vi "removeNode.vi"(0 "reference":refnum<class "Graph.lvclass">, 1 "node":refnum<class "AbstractNode.lvclass">, 2 "RemoveChildrenIfAny(False)":bool, 5 "error in (no error)":errorcluster) -> (14 "reference out":refnum<class "Graph.lvclass">, 19 "error out":errorcluster)   [LabVIEW 2016, in "Graph.lvclass"]
doc: "public void removeNode(Node n)"
uses:
  <resource>/Framework/Providers/Open_GDS/UML/Graph_class/Graph.lvclass
  <resource>/Framework/Providers/Open_GDS/UML/AbstractNode_class/AbstractNode.lvclass
  <resource>/Framework/Providers/Open_GDS/UML/PackageNode_class/PackageNode.lvclass
  C:/Program Files (x86)/National Instruments/LabVIEW 2016/resource/Framework/Providers/Open_GDS/UML/AbstractNode_class/AbstractNode.lvclass
  <resource>/Framework/Providers/Open_GDS/UML/AbstractEdge_class/AbstractEdge.lvclass
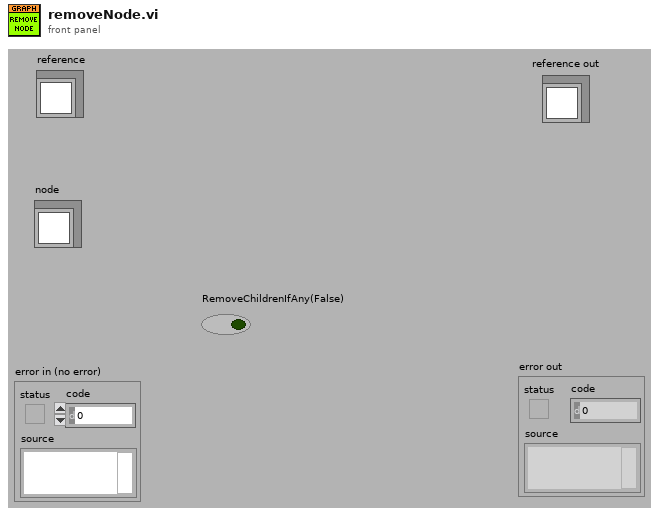
[diagram p1: front panel]
types:
  T1 = typedef "Graph.lvclass/ObjectAttributes.ctl" = cluster{"nodes":refnum<class "AbstractNode.lvclass">[], "edges":refnum<class "AbstractEdge.lvclass">[], "nodesToBeRemoved":refnum<class "AbstractNode.lvclass">[], "edgesToBeRemoved":refnum<class "AbstractEdge.lvclass">[], "needsLayout":bool, "LayoutNodes":refnum<class "AbstractNode.lvclass">[]}
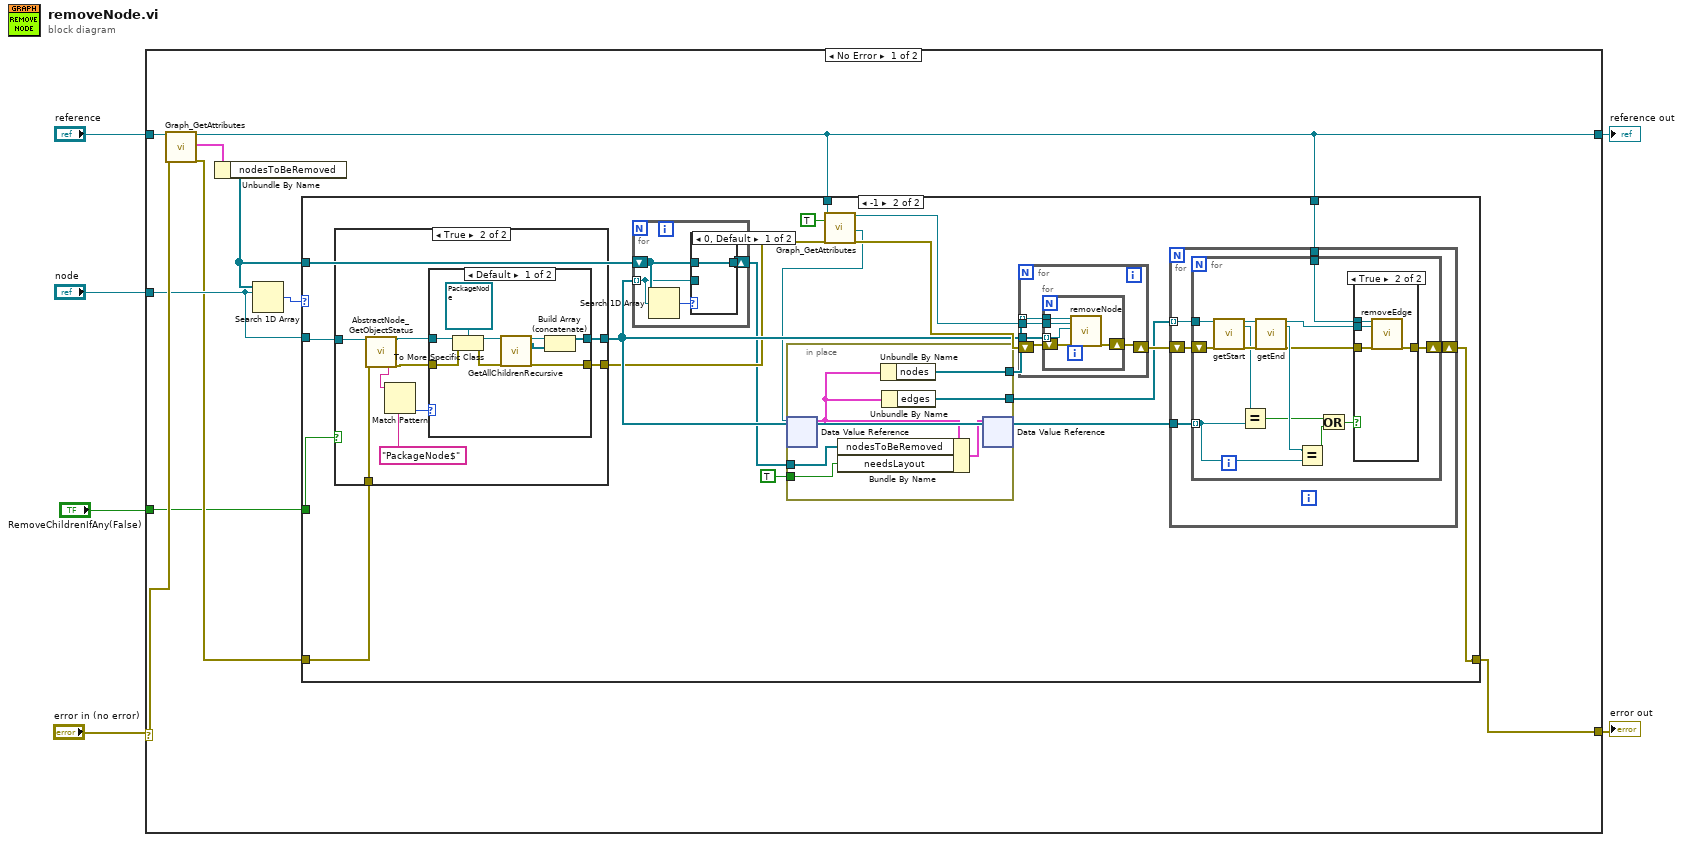
[diagram p0: block diagram]
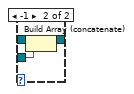
[diagram p3: hidden frame]
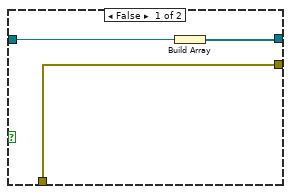
[diagram p4: hidden frame]
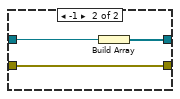
[diagram p5: hidden frame]
diagram:
  n1 = case shown="No Error" "error in (no error)" {
    selector: "error in (no error)" -> [w13 w108]
    tunnel: "reference" -> [w16 w109]
    tunnel: [w15 w108] -> w5
    tunnel: [w14 w109] -> w4
    tunnel: "node" -> [w12 _]
    tunnel: "RemoveChildrenIfAny(False)" -> [w8 _]
    frame No Error {
      n2 = call <resource>:"Graph_GetAttributes.vi"("reference in"=w16, "error in (no error)"=w13) -> ("reference out"=w14:refnum<class "Graph.lvclass">, "Data"=w7:T1, "error out"=w10:errorcluster)  [unwired: 1 in, 14 out]
      n3 = Unbundle By Name(w7) -> ("nodesToBeRemoved"=w9:refnum<class "AbstractNode.lvclass">[])
      n4 = Search 1D Array(1D array=w9, element=w12) -> (index of element=w11:i32)  [unwired: 1 out]
      n5 = case shown="-1" w11 {
        tunnel: w10 -> [w17 w26]
        tunnel: [w17 w30] -> w15
        tunnel: w14 -> [_ w35]
        tunnel: w9 -> [_ w34]
        tunnel: w12 -> [_ w27]
        tunnel: w14 -> [_ w29]
        tunnel: w8 -> [_ w24]
        frame 0, Default {
        }
        frame -1 {
          n6 = case shown="True" w24 {
            tunnel: [w51 w61] -> w28
            tunnel: w27 -> [w52 w60]
            tunnel: w26 -> [w50 w59]
            tunnel: [w50 w54] -> w25
            frame False {
              n7 = Build Array(w52) -> (w51:refnum<class "AbstractNode.lvclass">[])
            }
            frame True {
              n8 = call <resource>:"AbstractNode_GetObjectStatus.vi"("reference in"=w60, "error in (no error)"=w59) -> ("Class name"=w53:string, "reference out"=w56:refnum<class "AbstractNode.lvclass">, "error out"=w55:errorcluster)  [unwired: 15 out]
              n9 = Match Pattern(string=w53, regular expression="PackageNode$" ("y")) -> (offset past match=w57:i32)  [unwired: 4 out]
              n10 = case shown="Default" w57 {
                tunnel: [w62 w72] -> w54
                tunnel: [w63 w71] -> w61
                tunnel: w56 -> [w70 w73]
                tunnel: w55 -> [w68 w72]
                frame Default {
                  n11 = To More Specific Class(target class=refnum<class "PackageNode.lvclass"> refnum ("reference in"), reference=w70, error in=w68) -> (specific class reference=w66:refnum<class "PackageNode.lvclass">, error out=w67:errorcluster)
                  n12 = call <resource>:"GetAllChildrenRecursive.vi"("reference"=w66, "error in (no error)"=w67) -> ("reference out"=w65:refnum<class "PackageNode.lvclass">, "children"=w64:refnum<class "AbstractNode.lvclass">[], "error out"=w62:errorcluster)  [unwired: 15 in]
                  n13 = Build Array (concatenate)(w65, w64) -> (w63:refnum<class "AbstractNode.lvclass">[])
                }
                frame -1 {
                  n14 = Build Array(w73) -> (w71:refnum<class "AbstractNode.lvclass">[])
                }
              }
            }
          }
          n15 = for {
            tunnel: w28 -> [w42] mode=indexing
            shift-right: [w45] -> w19
            shift-left: w34 -> [w44]
            n16 = Search 1D Array(1D array=w44, element=w42) -> (index of element=w43:i32)  [unwired: 1 out]
            n17 = case shown="0, Default" w43 {
              tunnel: [w46 w49] -> w45
              tunnel: w42 -> [_ w48]
              tunnel: w44 -> [w46 w47]
              frame 0, Default {
              }
              frame -1 {
                n18 = Build Array (concatenate)(w47, w48) -> (w49:refnum<class "AbstractNode.lvclass">[])
              }
            }
          }
          n19 = call <resource>:"Graph_GetAttributes.vi"("reference in"=w35, "OnlyGetDvrReference(False)"=TRUE, "error in (no error)"=w25) -> ("reference out"=w33:refnum<class "Graph.lvclass">, "DataRef"=w22:refnum<data-value>, "error out"=w32:errorcluster)  [unwired: 13 in, 1 out]
          n20 = in-place {
            in-place-border: [w40] -> w21
            in-place-border: [w39] -> w20
            in-place-border: w19 -> [w38]
            in-place-border: TRUE ("needsLayout") -> [w37]
            n21 = in-place-dvr #1(w22) -> (w41:T1)  [unwired: 1 out]
            n22 = Bundle By Name(cluster=w41, "nodesToBeRemoved"=w38, "needsLayout"=w37) -> (w36:T1)
            n23 = Unbundle By Name(w41) -> ("nodes"=w40:refnum<class "AbstractNode.lvclass">[])
            n24 = Unbundle By Name(w41) -> ("edges"=w39:refnum<class "AbstractEdge.lvclass">[])
            n25 = in-place-dvr #1(w36) -> ()  [unwired: 2 out]
          }
          n26 = for {
            tunnel: w21 -> [w102] mode=indexing
            tunnel: w33 -> [w101]
            tunnel: w28 -> [w100]
            shift-right: [w98] -> w31
            shift-left: w32 -> [w99]
            n27 = for {
              tunnel: w102 -> [w107]
              tunnel: w101 -> [w106]
              tunnel: w100 -> [w103] mode=indexing
              shift-right: [w104] -> w98
              shift-left: w99 -> [w105]
              n28 = call-dynamic "removeNode.vi"("reference"=w107, "graph"=w106, "node"=w103, "error in (no error)"=w105) -> ("error out"=w104:errorcluster)  [unwired: 14 in, 1 out]
            }
          }
          n29 = for {
            tunnel: w20 -> [w77] mode=indexing
            shift-right: [w75] -> w30
            shift-left: w31 -> [w78]
            tunnel: w28 -> [w76]
            tunnel: w29 -> [w74]
            n30 = for {
              tunnel: w77 -> [w91]
              tunnel: w76 -> [w86] mode=indexing
              tunnel: w74 -> [w80]
              shift-right: [w83] -> w75
              shift-left: w78 -> [w92]
              n31 = call-dynamic "getStart.vi"("reference"=w91, "error in (no error)"=w92) -> ("reference out"=w90:refnum<class "AbstractEdge.lvclass">, "startNode"=w88:refnum<class "AbstractNode.lvclass">, "error out"=w89:errorcluster)  [unwired: 14 in, 1 out]
              n32 = Equal?(x=w88, y=w86) -> (x = y?=w84:bool)
              n33 = call-dynamic "getEnd.vi"("reference"=w90, "error in (no error)"=w89) -> ("reference out"=w79:refnum<class "AbstractEdge.lvclass">, "endNode"=w87:refnum<class "AbstractNode.lvclass">, "error out"=w82:errorcluster)  [unwired: 14 in, 1 out]
              n34 = Equal?(x=w87, y=w86) -> (x = y?=w85:bool)
              n35 = Or(x=w84, y=w85) -> (x .or. y?=w81:bool)
              n36 = case shown="True" w81 {
                tunnel: [w93 w97] -> w83
                tunnel: w82 -> [w93 w96]
                tunnel: w80 -> [_ w95]
                tunnel: w79 -> [_ w94]
                frame False {
                }
                frame True {
                  n37 = call-dynamic "removeEdge.vi"("reference"=w95, "edge"=w94, "error in (no error)"=w96) -> ("error out"=w97:errorcluster)  [unwired: 15 in, 1 out]
                }
              }
            }
          }
        }
      }
    }
    frame Error {
    }
  }
  "reference out" <- w4
  "error out" <- w5
